vi "Update Status.vi"(8 "error in (no error)":errorcluster, 9 "Status":string, 10 "Name":string, 11 "Main In":refnum<class "Main.lvclass">) -> (0 "error out":errorcluster, 3 "Main Out":refnum<class "Main.lvclass">)   [LabVIEW 2020, in "Main.lvclass"]
uses:
  Main.lvclass
  Main.lvclass/Main.ctl
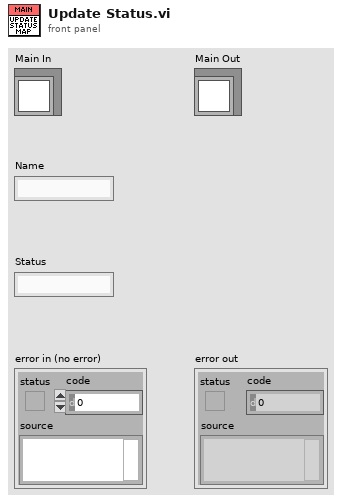
[diagram p1: front panel]
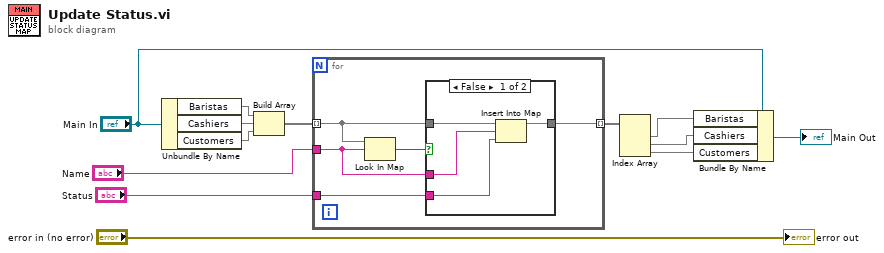
[diagram p0: block diagram]
diagram:
  n1 = Unbundle By Name("Main In") -> ("Baristas"=w11:map{string, string}, "Cashiers"=w10:map{string, string}, "Customers"=w9:map{string, string})
  n2 = Build Array(w11, w10, w9) -> (w8:map{string, string}[])
  n3 = for {
    tunnel: w8 -> [w18] mode=indexing
    tunnel: "Name" -> [w15]
    tunnel: [w17] -> w4 mode=indexing
    tunnel: "Status" -> [w14]
    n4 = Look In Map(map=w18, key=w15) -> (key not found?=w16:bool)  [unwired: 1 in, 1 out]
    n5 = case shown="False" w16 {
      tunnel: w18 -> [w22 w23]
      tunnel: [w21 w23] -> w17
      tunnel: w15 -> [w20 _]
      tunnel: w14 -> [w19 _]
      frame False {
        n6 = Insert Into Map(map in=w22, key=w20, value=w19) -> (map out=w21:map{string, string})  [unwired: 2 out]
      }
      frame True {
      }
    }
  }
  n7 = Index Array(array=w4) -> (element #1=w3:map{string, string}, element #2=w2:map{string, string}, element #3=w1:map{string, string})  [unwired: 3 in]
  n8 = Bundle By Name(cluster="Main In", "Baristas"=w3, "Cashiers"=w2, "Customers"=w1) -> (→"Main Out":refnum<class "Main.lvclass">)
  "error out" <- "error in (no error)"
